vi "Set Logging.vi"(11 "LogGroups":i32) -> (3 "function return":i32)   [LabVIEW 2025, in "ExtremelyEpicImagerIPC2.lvlib"]
doc: "IMAGERIPC_API HRESULT WINAPI SetLogging(int LogGroups);"
uses:
  ExtremelyEpicImagerIPC2.lvlib
  ImagerIPC2.dll
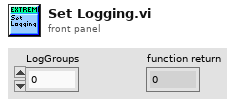
[diagram p1: front panel]
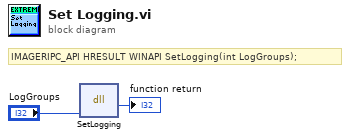
[diagram p0: block diagram]
diagram:
  # "IMAGERIPC_API HRESULT WINAPI SetLogging(int LogGroups);"
  n1 = dll-call lib="C:/Users/mayhe/OneDrive/Documents/GitHub/In-situ-monitoring-of-powder-bed-fusion-additive-manufacturing/system_development/Orichalcum/v0.2/Software_design/thermal-camera/VI/Connect SDK/ImagerIPC2.*" fn="SetLogging"("LogGroups"="LogGroups") -> (→"function return":i32)  [unwired: 4 in, 2 out]
